vi "Gyro Acc Dec Back Dis.vi"(4 "Stop rotation":i32=1200, 6 "Ini. Degrees":sgl, 7 "Motor":cluster{"Port":T2, "Port":T2}={"Port"=1, "Port"=2} {"Port" items=["Port A", "Port B", "Port C", "Port D"]; "Port" items=["Port A", "Port B", "Port C", "Port D"]}, 8 "Threshold to De-acc":i32=1000, 9 "De-acc":i32=40, 10 "Acc":i32=80, 11 "EV3 in":T1) -> (3 "EV3 out":T1)   [LabVIEW 2016]
uses:
  <vilib>/NXT/Block Support/NXT_OutputPort.ctl
  <vilib>/NXT/Subs/LVHSConnector.ctl
  <vilib>/NXT/LegoClasses/BrickReference/BrickReference.lvclass
  <vilib>/NXT/Block Support/NXT_InputPort.ctl
  <vilib>/NXT/NXTIO Xnodes/NXTIONodeSubVIs/LEGOResetMotors.vi
  <vilib>/NXT/Dual Mode Library/Motors/Rotation.vi
  <vilib>/NXT/Dual Mode Library/Sensors/EV3_Gyro_Angle.vi
  <vilib>/NXT/NXTIO Xnodes/NXTIONodeSubVIs/NXTMotorSteeringOn.vi
  <vilib>/NXT/NXTIO Xnodes/NXTIONodeSubVIs/NXTStopMotors.vi
  <vilib>/NXT/Dual Mode Library/Waits/Wait_Num.vi
  <vilib>/NXT/NXTIO Xnodes/NXTIOXNode/NXTIO.xnode
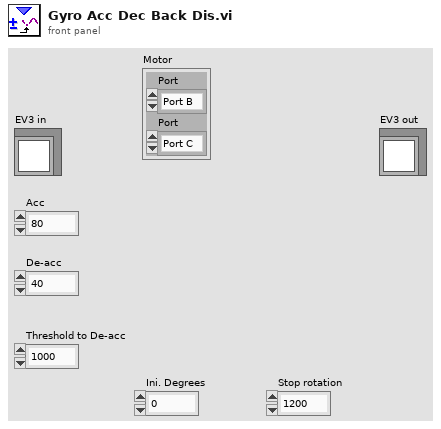
[diagram p1: front panel]
types:
  T1 = typedef "LVHSConnector.ctl" = refnum<class "BrickReference.lvclass">
  T2 = typedef "NXT_OutputPort.ctl" = u8
  T3 = typedef "NXT_InputPort.ctl" = u32
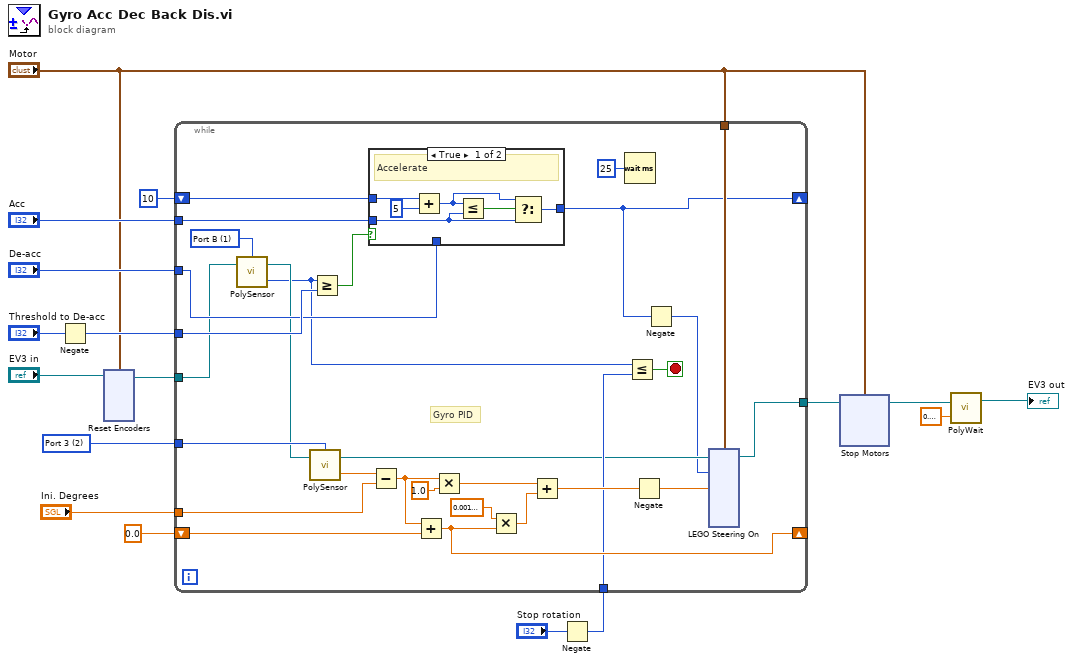
[diagram p0: block diagram]
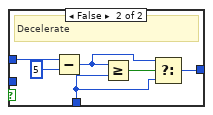
[diagram p2: hidden frame]
diagram:
  w15 = T3 2 items=["Port 1", "Port 2", "Port 3", "Port 4"] ("Port (Gyro)")
  n1 = Negate(x="Threshold to De-acc") -> (-x=w5:i32)
  n2 = xnode "Reset Encoders"("Motors"="Motor", "NXT/EV3"="EV3 in") -> ("NXT/EV3"=w12:T1)
  n3 = Negate(x="Stop rotation") -> (-x=w6:i32)
  n4 = while {
    tunnel: w12 -> [w27]
    tunnel: w15 -> [w35]
    shift-right: [w43] -> _
    shift-left: sgl 0.0 -> [w44]
    tunnel: "Ini. Degrees" -> [w39]
    tunnel: [w34] -> w8
    tunnel: "Motor" -> [w37]
    shift-right: [w19] -> _
    shift-left: 10 -> [w31]
    tunnel: "De-acc" -> [w28]
    tunnel: "Acc" -> [w30]
    tunnel: w5 -> [w29]
    tunnel: w6 -> [w22]
    stop <- w24 stop-if-true
    w36 = T2 1 items=["Port A", "Port B", "Port C", "Port D"] ("Port (Port A)")
    # "Gyro PID"
    n5 = call-poly <vilib>:"PolySensor.vi"("NXT/EV3"=w27, "Port (Port A)"=w36) -> ("Angle of Rotation"=w23:i32, "NXT/EV3"=w26:T1)  [unwired: 1 in]
    n6 = call-poly <vilib>:"PolySensor.vi"("NXT/EV3"=w26, "Port (Port 1)"=w35) -> ("Degrees"=w46:sgl, "NXT/EV3"=w21:T1)  [unwired: 1 in]
    n7 = Greater Or Equal?(x=w23, y=w29) -> (x >= y?=w25:bool)
    n8 = case shown="True" w25 {
      tunnel: w30 -> [w48 _]
      tunnel: w31 -> [w51 w57]
      tunnel: [w47 w54] -> w19
      tunnel: w28 -> [_ w53]
      frame True {
        # "Accelerate"
        n9 = Add(x=w51, y=5) -> (x+y=w49:i32)
        n10 = Less Or Equal?(x=w49, y=w48) -> (x <= y?=w50:bool)
        n11 = Select(t=w49, s=w50, f=w48) -> (s? t:f=w47:i32)
      }
      frame False {
        # "Decelerate"
        n12 = Subtract(x=w57, y=5) -> (x-y=w55:i32)
        n13 = Greater Or Equal?(x=w55, y=w53) -> (x >= y?=w56:bool)
        n14 = Select(t=w55, s=w56, f=w53) -> (s? t:f=w54:i32)
      }
    }
    n15 = Subtract(x=w46, y=w39) -> (x-y=w38:sgl)
    n16 = Add(x=w38, y=w44) -> (x+y=w43:sgl)
    n17 = Multiply(x=w38, y=sgl 1.0 ("K_p")) -> (x*y=w41:sgl)
    n18 = Multiply(x=sgl 0.001 ("K_i"), y=w43) -> (x*y=w40:sgl)
    n19 = Add(x=w41, y=w40) -> (x+y=w32:sgl)
    n20 = Wait (ms)(milliseconds to wait=u32 25) -> ()  [unwired: 1 out]
    n21 = Less Or Equal?(x=w23, y=w22) -> (x <= y?=w24:bool)
    n22 = Negate(x=w32) -> (-x=w18:sgl)
    n23 = Negate(x=w19) -> (-x=w20:i32)
    n24 = xnode "LEGO Steering On"("Steering 1"=w18, "Power 1"=w20, "Motors"=w37, "NXT/EV3"=w21) -> ("NXT/EV3"=w34:T1)
  }
  n25 = xnode "Stop Motors"("Motors"="Motor", "NXT/EV3"=w8) -> ("NXT/EV3"=w2:T1)
  n26 = call-poly <vilib>:"PolyWait.vi"("Time (1 sec)"=sgl 0.2, "NXT/EV3"=w2) -> ("NXT/EV3"=→"EV3 out":T1)  [unwired: 2 in]
